vi "Read Camera.vi"(9 "error in":errorcluster, 10 "Session In":T1) -> (0 "Frame Rate":dbl, 1 "error out":errorcluster, 2 "Session Out":T1, 3 "Image Out":T2(plugin-control))   [LabVIEW 2017]
uses:
  <vilib>/userdefined/High Color/IMAQdx.ctl
  <vilib>/vision/driver/NI_Vision_Acquisition_Software.lvlib
panel:
  out "Image Number":u32
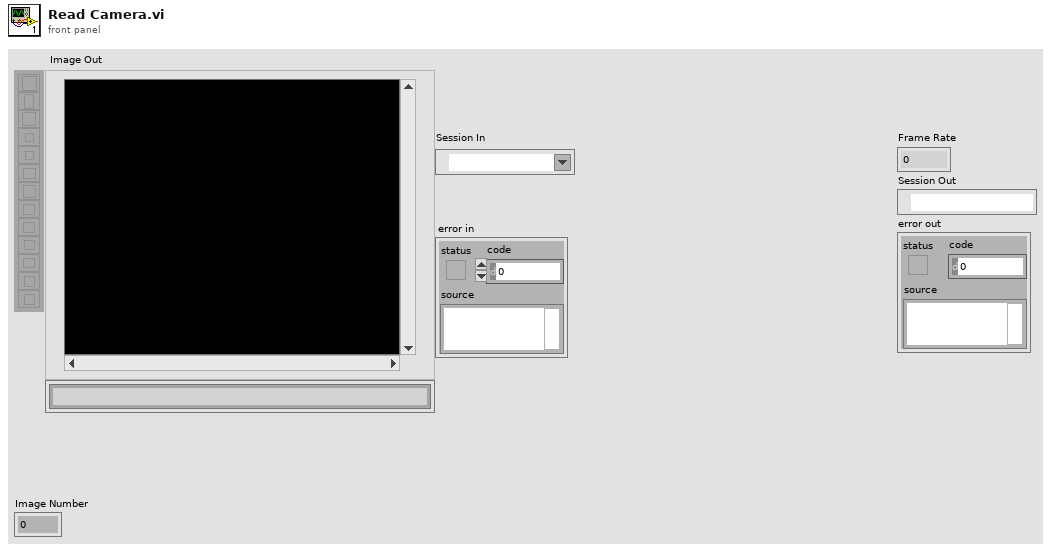
[diagram p1: front panel]
types:
  T1 = typedef "IMAQdx.ctl" = refnum<k21>
  T2 = typedef "IMAQ Image.ctl" = refnum<image>
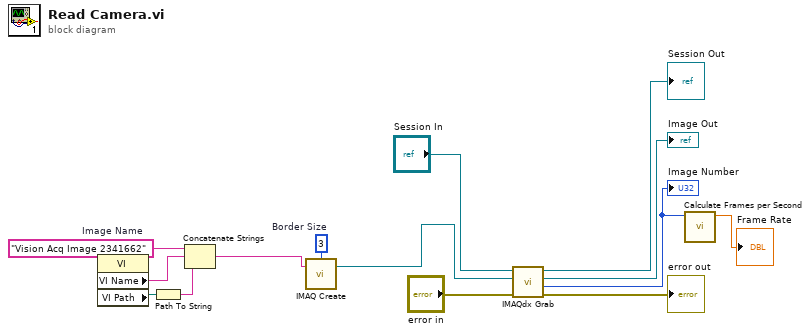
[diagram p0: block diagram]
diagram:
  w2 = 3  # Border Size
  w3 = "Vision Acq Image 2341662"  # Image Name
  n1 = property class="VI"() -> ("VI Name"=w6:string, "VI Path"=w7:path)  [unwired: 2 in, 2 out]
  n2 = Path To String(path=w7) -> (string=w5:string)
  n3 = Concatenate Strings(w3, w6, w5) -> (w4:string)
  n4 = call "IMAQ Create"("Border Size"=w2, "Image Name"=w4) -> ("New Image"=w1:T2)  [unwired: 2 in, 2 out]
  n5 = call <vilib>:"IMAQdx Grab.vi"("error in"="error in", "Image In"=w1, "Session In"="Session In") -> ("error out"=→"error out":errorcluster, "Buffer Number Out"=w13:u32, "Image Out"=→"Image Out":T2, "Session Out"=→"Session Out":T1)  [unwired: 1 in, 4 out]
  "Image Number" <- w13
  n6 = call <vilib>:"Calculate Frames per Second.vi"("Buffer Number"=w13) -> ("Acquired Frames/s"=→"Frame Rate":dbl)  [unwired: 2 in, 8 out]
